vi "dfd_Extract Output from I160.vi"(2 "I160":T2, 3 "output MSB pos":i16, 4 "Output wl":i16, 8 "q_mode":T1=enum."Truncation" caption="round mode") -> (7 "y":i32 format="%.0x")   [LabVIEW 2017, in "NI_DigFilter_FXP.lvlib"]
uses:
  <vilib>/addons/Digital Filter Design/NI_DigFilter_FXP.lvlib
  <vilib>/addons/Digital Filter Design/_Objects.llb/dfd_Integer I160.ctl
  <vilib>/addons/Digital Filter Design/_Objects.llb/DFD Round-off Mode.ctl
  <vilib>/addons/Digital Filter Design/NI_DigFilterLicensed.lvlib
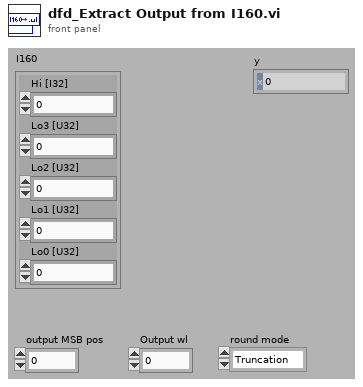
[diagram p1: front panel]
types:
  T1 = typedef "NI_DigFilterLicensed.lvlib/DFD Round-off Mode.ctl" = enum16{"Nearest", "Truncation"}
  T2 = typedef "dfd_Integer I160.ctl" = cluster{"Hi [I32]":i32, "Lo3 [U32]":u32, "Lo2 [U32]":u32, "Lo1 [U32]":u32, "Lo0 [U32]":u32}
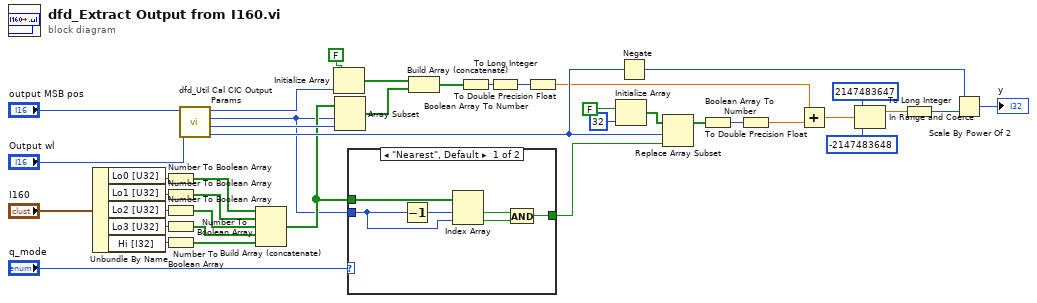
[diagram p0: block diagram]
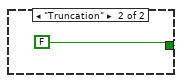
[diagram p2: hidden frame]
diagram:
  n1 = Unbundle By Name("I160") -> ("Lo0 [U32]"=w40:u32, "Lo1 [U32]"=w39:u32, "Lo2 [U32]"=w37:u32, "Lo3 [U32]"=w38:u32, "Hi [I32]"=w36:i32)
  n2 = Number To Boolean Array(number=w40) -> (Boolean array=w32:bool[])
  n3 = Number To Boolean Array(number=w39) -> (Boolean array=w31:bool[])
  n4 = Number To Boolean Array(number=w37) -> (Boolean array=w30:bool[])
  n5 = Number To Boolean Array(number=w38) -> (Boolean array=w29:bool[])
  n6 = Number To Boolean Array(number=w36) -> (Boolean array=w28:bool[])
  n7 = call <vilib>:"dfd_Util Cal CIC Output Params.vi"("Output wl"="Output wl", "output MSB pos"="output MSB pos") -> ("Shift"=w12:i16, "length"=w25:i16, "index"=w2:i16, "zero padding"=w21:i16)  [unwired: 6 out]
  n8 = Build Array (concatenate)(w32, w31, w30, w29, w28) -> (w3:bool[])
  n9 = Initialize Array(FALSE, w21) -> (w22:bool[])
  n10 = Array Subset(array=w3, index=w2, length=w25) -> (w23:bool[])
  n11 = case shown="\"Nearest\", Default" "q_mode" {
    tunnel: [w45 FALSE] -> w17
    tunnel: w3 -> [w43 _]
    tunnel: w2 -> [w42 _]
    frame "Nearest", Default {
      n12 = Decrement(x=w42) -> (x-1=w44:i16)
      n13 = Index Array(array=w43, index #1=w44, index #2=w42) -> (element #1=w46:bool, element #2=w41:bool)
      n14 = And(x=w46, y=w41) -> (x .and. y?=w45:bool)
    }
    frame "Truncation" {
    }
  }
  n15 = Build Array (concatenate)(w22, w23) -> (w20:bool[])
  n16 = Boolean Array To Number(Boolean array=w20) -> (number=w34:u32)
  n17 = To Long Integer(number=w34) -> (32bit integer=w11:i32)
  n18 = To Double Precision Float(number=w11) -> (double precision float=w9:dbl)
  n19 = Initialize Array(FALSE, 32 ("dimension size")) -> (w14:bool[])
  n20 = Negate(x=w12) -> (-x=w15:i16)
  n21 = Replace Array Subset(array=w14, new element=w17, index=w12) -> (w16:bool[])
  n22 = Boolean Array To Number(Boolean array=w16) -> (number=w1:u32)
  n23 = To Double Precision Float(number=w1) -> (double precision float=w10:dbl)
  n24 = Add(x=w9, y=w10) -> (x+y=w8:dbl)
  n25 = In Range and Coerce(upper limit=2147483647, x=w8, lower limit=-2147483648) -> (coerced(x)=w5:dbl)  [unwired: 1 out]
  n26 = To Long Integer(number=w5) -> (32bit integer=w4:i32)
  n27 = Scale By Power Of 2(n=w15, x=w4) -> (x*2^n=→"y":i32)
